vi "comand to array bool.vi"(11 "Command to Send":string="SRC012;") -> (2 "Puerto":string, 3 "output array":bool[](array[boolean]))   [LabVIEW 2020, in "Test simulado.lvclass"]
uses:
  Test simulado.lvclass
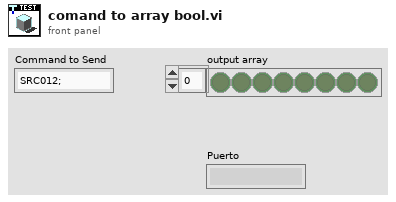
[diagram p1: front panel]
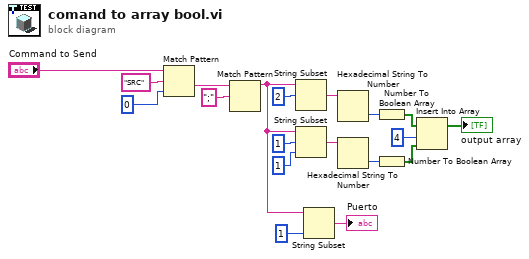
[diagram p0: block diagram]
diagram:
  n1 = Match Pattern(string="Command to Send", regular expression="SRC" ("string"), offset (0)=0) -> (after substring=w16:string)  [unwired: 3 out]
  n2 = Match Pattern(string=w16, regular expression=";") -> (before substring=w3:string)  [unwired: 1 in, 3 out]
  n3 = String Subset(string=w3, offset (0)=2) -> (substring=w10:string)  [unwired: 1 in]
  n4 = String Subset(string=w3, offset (0)=1, length (rest)=1 ("length (rest)")) -> (substring=w9:string)
  n5 = String Subset(string=w3, length (rest)=1 ("length (rest)")) -> (substring=→"Puerto":string)  [unwired: 1 in]
  n6 = Hexadecimal String To Number(string=w10) -> (number=w8:u32)  [unwired: 2 in, 1 out]
  n7 = Hexadecimal String To Number(string=w9) -> (number=w7:u32)  [unwired: 2 in, 1 out]
  n8 = Number To Boolean Array(number=w8) -> (Boolean array=w4:bool[])
  n9 = Number To Boolean Array(number=w7) -> (Boolean array=w5:bool[])
  n10 = Insert Into Array(array=w4, index=4, new element=w5) -> (→"output array":bool[])
